vi "Connect PV.vi"(8 "error in (no error)":errorcluster, 10 "PV URL":string, 11 "CS++SVMonitor in":refnum<class "CS++SVMonitor.lvclass">) -> (0 "error out":errorcluster, 3 "CS++SVMonitor out":refnum<class "CS++SVMonitor.lvclass">)   [LabVIEW 2013, in "CS++SVMonitor.lvlib" / "CS++SVMonitor.lvclass"]
doc: "Open connection to process variable."
uses:
  CS++SVMonitor.lvclass
  CS++SVMonitor.lvclass/CS++SVMonitor.ctl
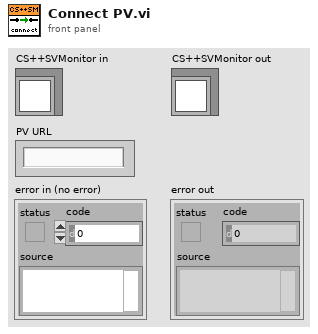
[diagram p1: front panel]
types:
  T1 = cluster{"Read Access":enum8{"Allowed", "Required", "None"}, "Write Access":enum8{"Allowed", "Required", "None"}}
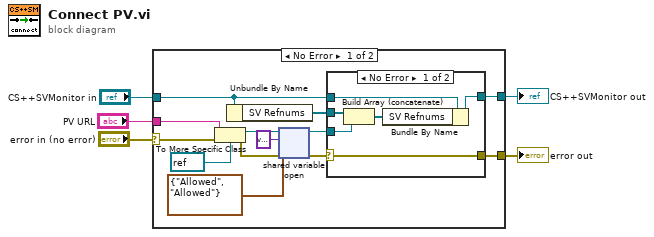
[diagram p0: block diagram]
diagram:
  n1 = case shown="No Error" "error in (no error)" {
    selector: "error in (no error)" -> [w12 w28]
    tunnel: [w6 w28] -> w2
    tunnel: [w9 w27] -> w3
    tunnel: "CS++SVMonitor in" -> [w10 w27]
    tunnel: "PV URL" -> [w11 _]
    frame No Error {
      n2 = To More Specific Class(target class=refnum<k21> refnum ("shared variable refnum in"), reference=w11, error in=w12) -> (specific class reference=w17:refnum<k21>, error out=w16:errorcluster)
      n3 = Unbundle By Name(w10) -> ("SV Refnums"=w8:refnum<k21>[])
      n4 = shared-variable-open(w17, w16, variant ("variant"), T1 {"Read Access"=enum."Allowed", "Write Access"=enum."Allowed"} ("access")) -> (w13:refnum<k21>, w7:errorcluster)
      n5 = case shown="No Error" w7 {
        selector: w7 -> [w19 w25]
        tunnel: w13 -> [w24 _]
        tunnel: w10 -> [w23 w26]
        tunnel: [w22 w26] -> w9
        tunnel: w8 -> [w20 _]
        tunnel: [w19 w25] -> w6
        frame No Error {
          n6 = Build Array (concatenate)(w20, w24) -> (w21:refnum<k21>[])
          n7 = Bundle By Name(cluster=w23, "SV Refnums"=w21) -> (w22:refnum<class "CS++SVMonitor.lvclass">)
        }
        frame Error {
        }
      }
    }
    frame Error {
    }
  }
  "error out" <- w2
  "CS++SVMonitor out" <- w3
